vi "Initialize Color Processors.vi"(8 "error in (no error)":errorcluster, 9 "Camera Color Correction Matrix":sgl[](array[numeric]), 10 "White Balance Matrix":sgl[](array[numeric]), 11 "BitDepth":i32) -> (0 "error out":errorcluster, 3 "Color Processor References":T1)   [LabVIEW 2015]
uses:
  C:/code/ScientificCameraInterfaces/Installer/Scientific Camera Interfaces/LabVIEW/64_bit/Library_X64/Thorlabs.TSI.Demosaicker.dll
  code/ScientificCameraInterfaces/Installer/Scientific Camera Interfaces/LabVIEW/64_bit/Library_X64/Thorlabs.TSI.Demosaicker.dll
  C:/code/ScientificCameraInterfaces/Installer/Scientific Camera Interfaces/LabVIEW/64_bit/Library_X64/Thorlabs.TSI.ColorProcessor.dll
  code/ScientificCameraInterfaces/Installer/Scientific Camera Interfaces/LabVIEW/64_bit/Library_X64/Thorlabs.TSI.ColorProcessor.dll
  C:/code/ScientificCameraInterfaces/Installer/Scientific Camera Interfaces/LabVIEW/64_bit/Library_X64/Thorlabs.TSI.ColorInterfaces.dll
  code/ScientificCameraInterfaces/Installer/Scientific Camera Interfaces/LabVIEW/64_bit/Library_X64/Thorlabs.TSI.ColorInterfaces.dll
  Color/Color Processor References.ctl
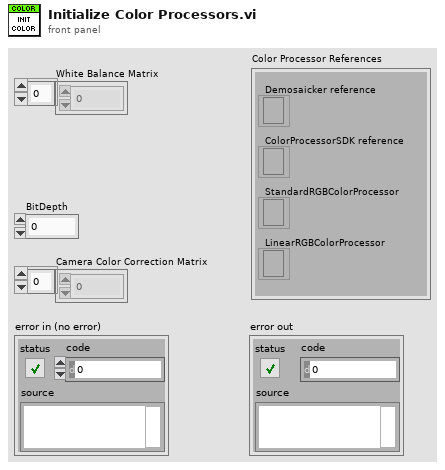
[diagram p1: front panel]
types:
  T1 = typedef "Color Processor References.ctl" = cluster{"Demosaicker reference":refnum<k24>, "ColorProcessorSDK reference":refnum<k24>, "StandardRGBColorProcessor":refnum<k24>, "LinearRGBColorProcessor":refnum<k24>}
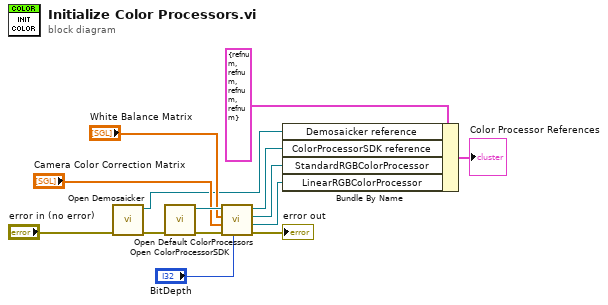
[diagram p0: block diagram]
diagram:
  n1 = call "Open Demosaicker.vi"("error in (no error)"="error in (no error)") -> ("error out"=w7:errorcluster, "Demosaicker reference"=w6:refnum<k24>)  [unwired: 9 in]
  n2 = call "Open ColorProcessorSDK.vi"("error in (no error)"=w7) -> ("error out"=w8:errorcluster, "ColorProcessorSDK reference"=w12:refnum<k24>)  [unwired: 9 in]
  n3 = call "Open Default ColorProcessors.vi"("Bit Depth"="BitDepth", "error in (no error)"=w8, "Color Correction Matrix"="Camera Color Correction Matrix", "White Balance Matrix"="White Balance Matrix", "ColorProcessorSDK reference"=w12) -> ("error out"=→"error out":errorcluster, "LinearRGBColorProcessor"=w3:refnum<k24>, "StandardRGBColorProcessor"=w4:refnum<k24>, "ColorProcessorSDK reference out"=w5:refnum<k24>)  [unwired: 3 in]
  n4 = Bundle By Name(cluster=T1 {"Demosaicker reference"=refnum, "ColorProcessorSDK reference"=refnum, "StandardRGBColorProcessor"=refnum, "LinearRGBColorProcessor"=refnum} ("Color Processor References"), "Demosaicker reference"=w6, "ColorProcessorSDK reference"=w5, "StandardRGBColorProcessor"=w4, "LinearRGBColorProcessor"=w3) -> (→"Color Processor References":T1)
